vi "Heat Up Macro Remove Parentheses.vi"(11 "Input Array":string[](array[string])) -> (3 "Clean Array":string[](array[string]))   [LabVIEW 2016]
uses:
  <vilib>/Utility/error.llb/whitespace.ctl
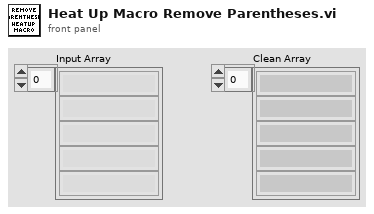
[diagram p1: front panel]
types:
  T1 = typedef "whitespace.ctl" = u16
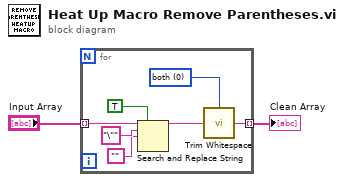
[diagram p0: block diagram]
diagram:
  n1 = for {
    tunnel: "Input Array" -> [w9] mode=indexing
    tunnel: [w3] -> w2 mode=indexing
    w4 = T1 0 items=["both", "start of string", "end of string"] ("location (both)")
    n2 = Search and Replace String(replace all?=TRUE ("replace all? (F)"), input string=w9, search string="\"", replace string="") -> (result string=w5:string)  [unwired: 4 in, 3 out]
    n3 = call <vilib>:"Trim Whitespace.vi"("string"=w5, "location (both)"=w4) -> ("trimmed string"=w3:string)
  }
  "Clean Array" <- w2
